vi "Data Out_Main.vi"(8 "error in":errorcluster, 11 "QRD":T1) -> (0 "error out":errorcluster)   [LabVIEW 2025]
uses:
  Controls/Queues-Refs-Data.ctl
  Builds/Queue Wrappers.lvlibp/Q Packet.ctl
  Controls/Acquisition Packet.ctl
  Builds/Queue Wrappers.lvlibp
  Controls/Local Data_Data Out.ctl
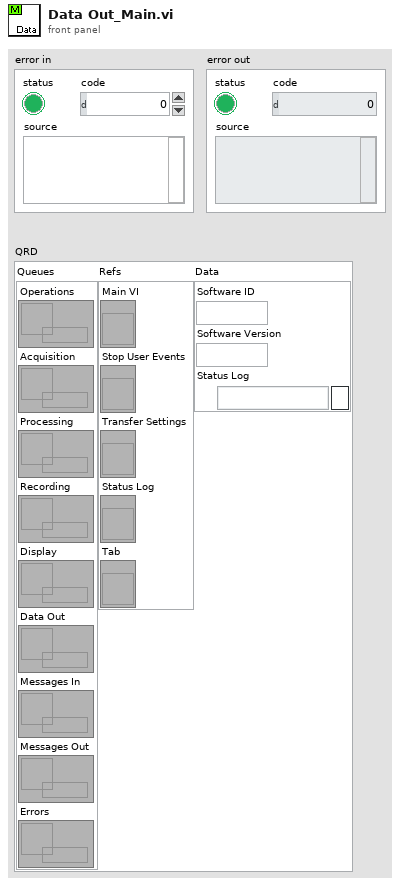
[diagram p1: front panel]
types:
  T1 = typedef "Queues-Refs-Data.ctl" = cluster{"Queues":cluster{"Operations":refnum<queue>, "Acquisition":refnum<queue>, "Processing":refnum<queue>, "Recording":refnum<queue>, "Display":refnum<queue>, "Data Out":refnum<queue>, "Messages In":refnum<queue>, "Messages Out":refnum<queue>, "Errors":refnum<queue>}, "Refs":cluster{"Main VI":refnum<vi>, "Stop User Events":refnum<vi>, "Transfer Settings":refnum<vi>, "Status Log":refnum<vi>, "Tab":refnum<vi>}, "Data":cluster{"Software ID":string, "Software Version":string, "Status Log":path}}
  T2 = typedef "Local Data_Data Out.ctl" = cluster{"Loop ID":string}
  T3 = typedef "Acquisition Packet.ctl" = cluster{"Time Stamp":timestamp, "Raw Data":cluster{"String":string, "Numeric":dbl, "Boolean":bool}, "Derived Data":cluster{"String":string, "Numeric":dbl, "Boolean":bool}}
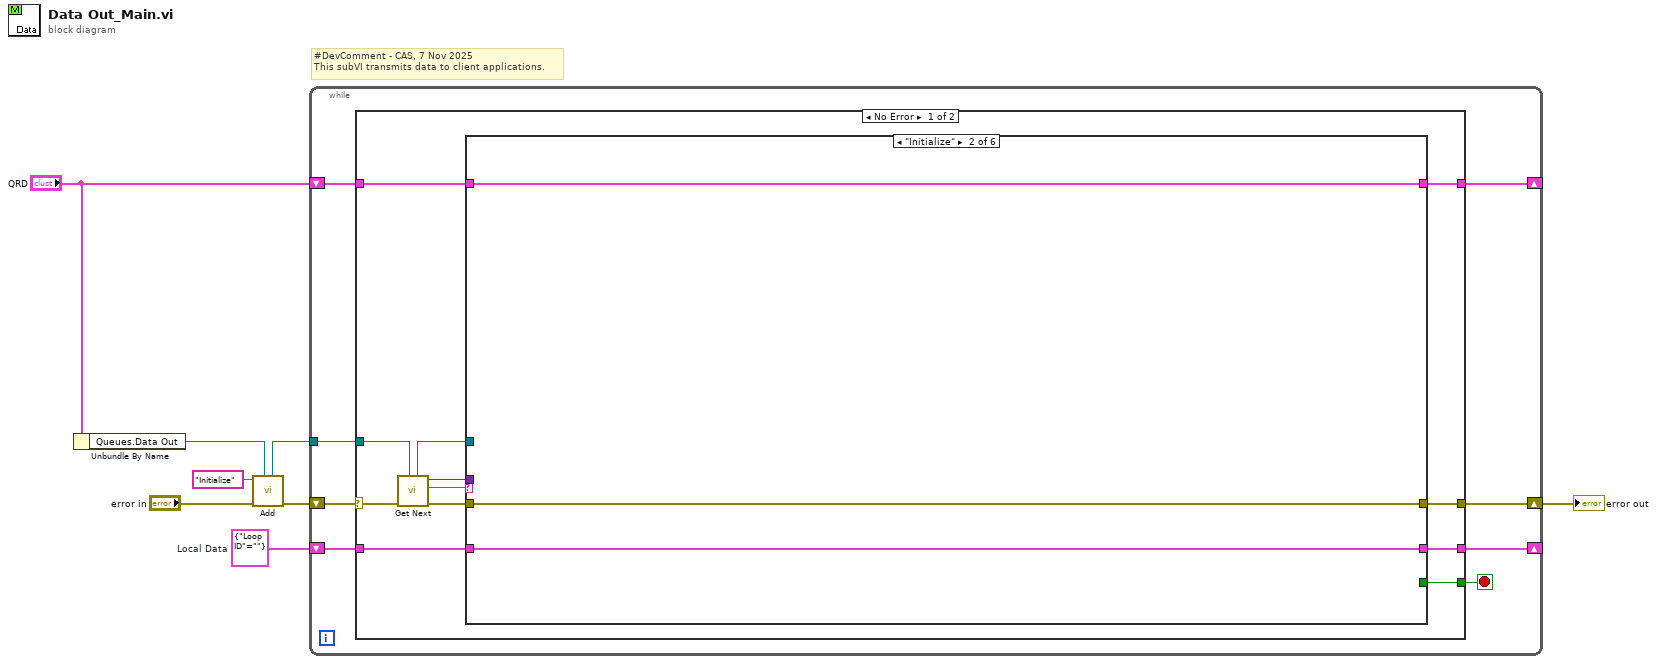
[diagram p0: block diagram]
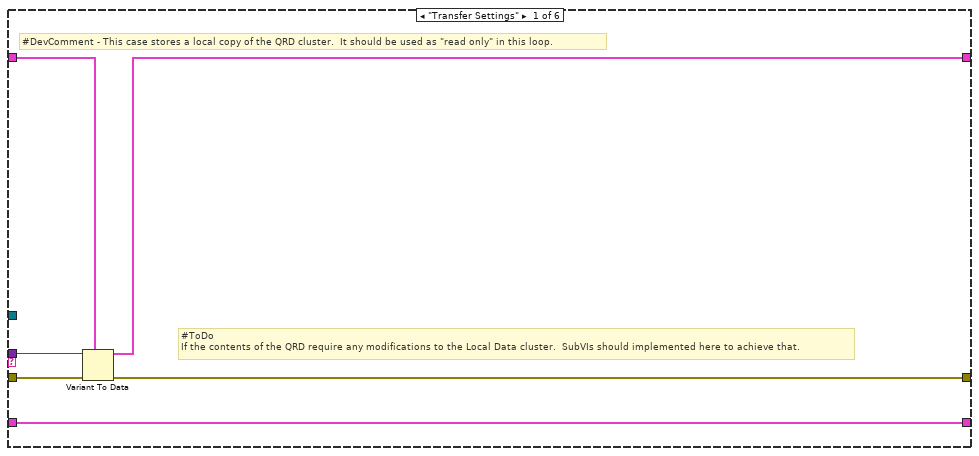
[diagram p2: hidden frame]
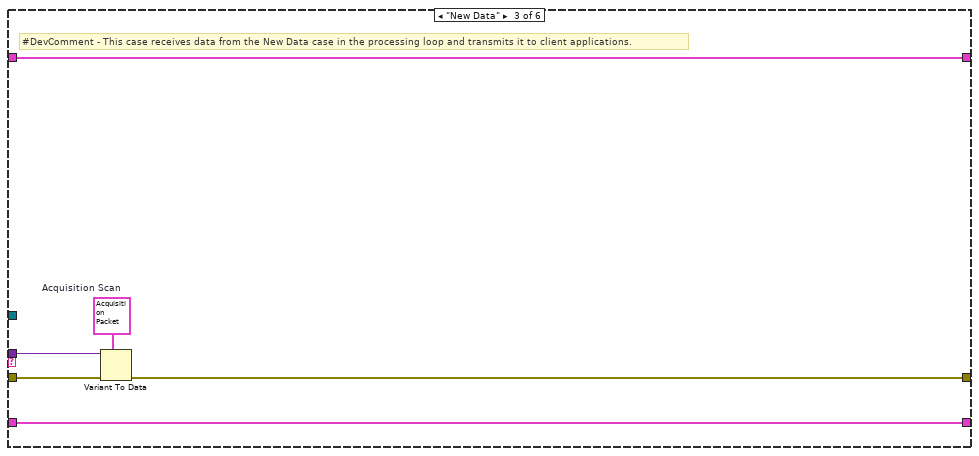
[diagram p3: hidden frame]
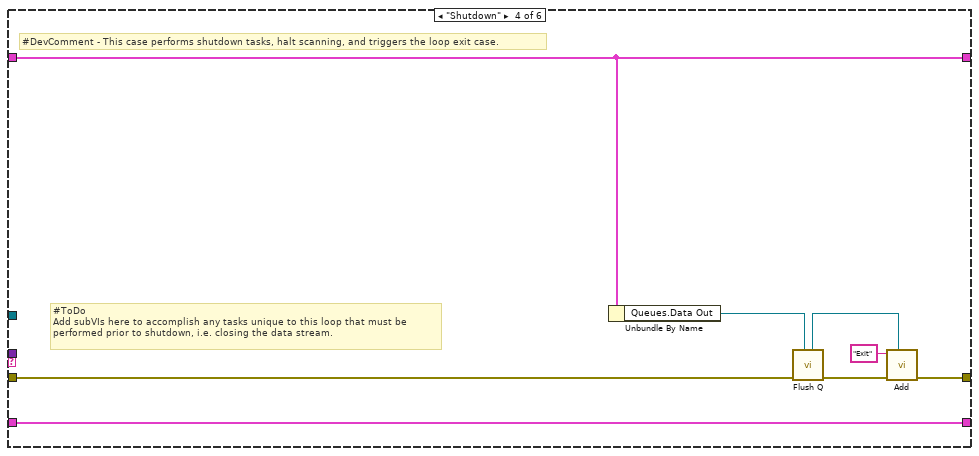
[diagram p4: hidden frame]
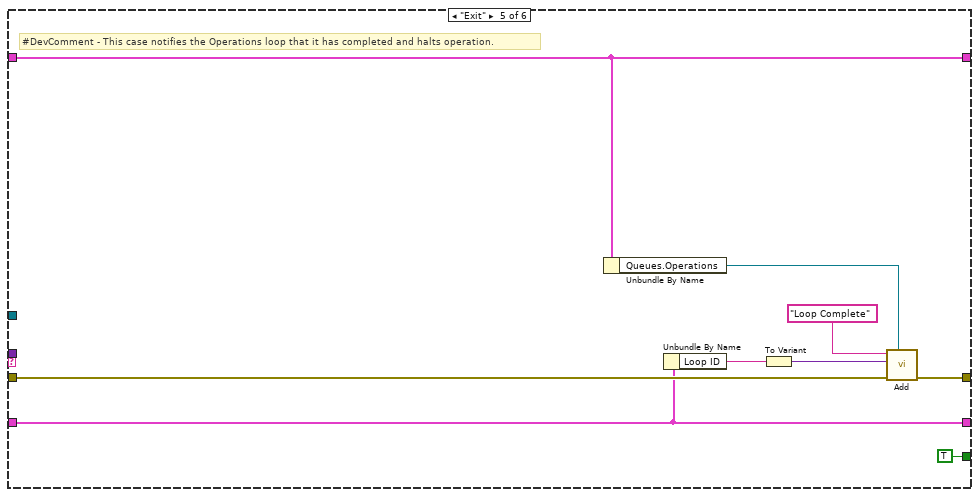
[diagram p5: hidden frame]
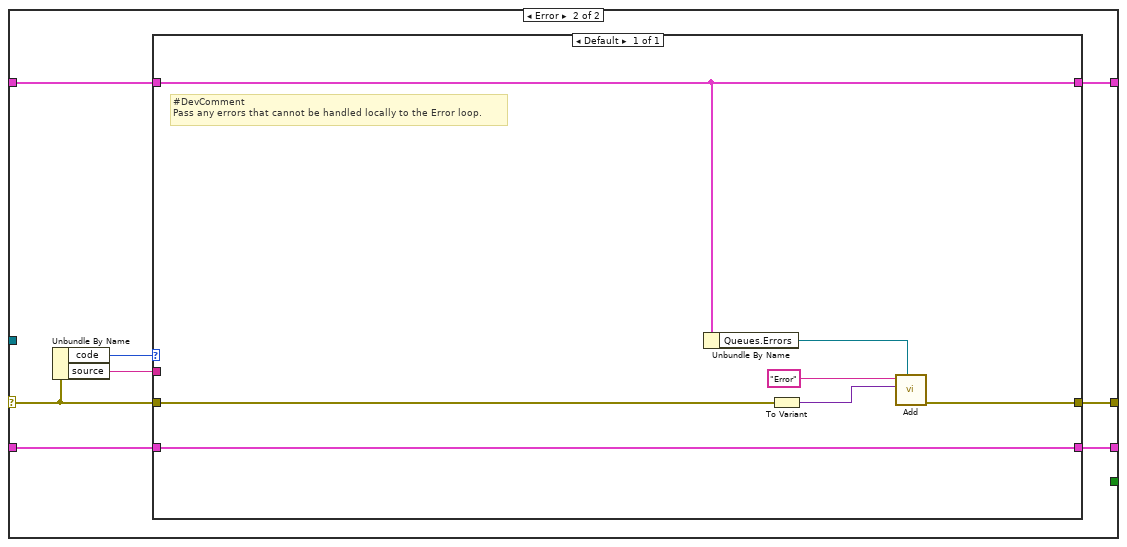
[diagram p7: hidden frame]
diagram:
  w6 = T2 {"Loop ID"=""}  # Local Data
  # "#DevComment - CAS, 7 Nov 2025\nThis subVI transmits data to client applications."
  n1 = Unbundle By Name("QRD") -> ("Queues.Data Out"=w3:refnum<queue>)
  n2 = call "Add.vi"("Q Ref In"=w3, "error in"="error in", "Packet ID"="Initialize") -> ("error out"=w4:errorcluster, "Q Ref Out"=w2:refnum<queue>)  [unwired: 5 in, 2 out]
  n3 = while {
    shift-right: [w15] -> _
    shift-left: "QRD" -> [w16]
    shift-right: [w13] -> w8
    shift-left: w4 -> [w14]
    tunnel: w2 -> [w12]
    shift-right: [w9] -> _
    shift-left: w6 -> [w11]
    stop <- w10 stop-if-true
    n4 = case shown="No Error" w14 {
      selector: w14 -> [w28 w68]
      tunnel: w16 -> [w25 w65]
      tunnel: [w26 w66] -> w15
      tunnel: [w23 w67] -> w13
      tunnel: w12 -> [w27 _]
      tunnel: w11 -> [w19 w69]
      tunnel: [w18 w64] -> w9
      tunnel: [w17 _] -> w10
      frame No Error {
        n5 = call "Get Next.vi"("Q Ref In"=w27, "error in"=w28) -> ("error out"=w24:errorcluster, "Packet ID"=w20:string, "Payload"=w21:variant, "Q Ref Out"=w22:refnum<queue>)  [unwired: 6 in]
        n6 = case shown="\"Initialize\"" w20 {
          tunnel: [w30 w37 w38 w51 w60 w63] -> w26
          tunnel: w25 -> [w32 w37 w38 w51 w60 w63]
          tunnel: w24 -> [w34 w36 w43 w48 w57 w62]
          tunnel: [w31 w36 w40 w50 w59 w62] -> w23
          tunnel: w22 -> [_ _ _ _ _ _]
          tunnel: w21 -> [w33 _ w42 _ _ _]
          tunnel: w19 -> [w29 w35 w39 w44 w55 w61]
          tunnel: [w29 w35 w39 w44 w55 w61] -> w18
          tunnel: [_ _ _ _ TRUE _] -> w17
          frame "Transfer Settings" {
            # "#ToDo\nIf the contents of the QRD require any modifications to the Local Data cluster.  SubVIs should implemented here to achieve that."
            # "#DevComment - This case stores a local copy of the QRD cluster.  It should be used as \"read only\" in this loop."
            n7 = Variant To Data(error in=w34, type=w32, Variant=w33) -> (data=w30:T1, error out=w31:errorcluster)
          }
          frame "Initialize" {
          }
          frame "New Data" {
            w41 = T3 {"Time Stamp"=timestamp(0 s since 1904-01-01), "Raw Data"={"String"="", "Numeric"=0.0, "Boolean"=FALSE}, "Derived Data"={"String"="", "Numeric"=0.0, "Boolean"=FALSE}}  # Acquisition Scan
            # "#DevComment - This case receives data from the New Data case in the processing loop and transmits it to client applications."
            n8 = Variant To Data(error in=w43, type=w41, Variant=w42) -> (error out=w40:errorcluster)  [unwired: 1 out]
          }
          frame "Shutdown" {
            # "#ToDo\nAdd subVIs here to accomplish any tasks unique to this loop that must be\nperformed prior to shutdown, i.e. closing the data stream."
            # "#DevComment - This case performs shutdown tasks, halt scanning, and triggers the loop exit case."
            n9 = Unbundle By Name(w51) -> ("Queues.Data Out"=w46:refnum<queue>)
            n10 = call "Flush Q.vi"("Q Ref In"=w46, "error in"=w48) -> ("error out"=w47:errorcluster, "Q Ref Out"=w45:refnum<queue>)  [unwired: 8 in]
            n11 = call "Add.vi"("Q Ref In"=w45, "error in"=w47, "Packet ID"="Exit") -> ("error out"=w50:errorcluster)  [unwired: 5 in, 3 out]
          }
          frame "Exit" {
            # "#DevComment - This case notifies the Operations loop that it has completed and halts operation."
            n12 = Unbundle By Name(w60) -> ("Queues.Operations"=w56:refnum<queue>)
            n13 = Unbundle By Name(w55) -> ("Loop ID"=w54:string)
            n14 = To Variant(anything=w54) -> (Variant=w53:variant)
            n15 = call "Add.vi"("Q Ref In"=w56, "error in"=w57, "Payload"=w53, "Packet ID"="Loop Complete") -> ("error out"=w59:errorcluster)  [unwired: 4 in, 3 out]
          }
          frame Default {
          }
        }
      }
      frame Error {
        n16 = Unbundle By Name(w68) -> ("code"=w71:i32, "source"=w70:string)
        n17 = case shown="Default" w71 {
          tunnel: w70 -> [_]
          tunnel: w69 -> [w78]
          tunnel: [w78] -> w64
          tunnel: w68 -> [w73]
          tunnel: [w75] -> w67
          tunnel: [w74] -> w66
          tunnel: w65 -> [w74]
          frame Default {
            # "#DevComment\nPass any errors that cannot be handled locally to the Error loop."
            n18 = Unbundle By Name(w74) -> ("Queues.Errors"=w76:refnum<queue>)
            n19 = To Variant(anything=w73) -> (Variant=w72:variant)
            n20 = call "Add.vi"("Q Ref In"=w76, "Payload"=w72, "Packet ID"="Error") -> ("error out"=w75:errorcluster)  [unwired: 5 in, 3 out]
          }
        }
      }
    }
  }
  "error out" <- w8
